vi "multipliers.vi"(7 "LabVIEW Web Service Request":refnum<class "Web Request.lvclass">, 11 "mult":string) -> ()   [LabVIEW 2014]
uses:
  <vilib>/wsapi/Web Request.lvclass
  Controller/Controller.lvclass
  Controller/Messages/Update TE Tech Heating Params/Update TE Tech Heating Params.lvclass
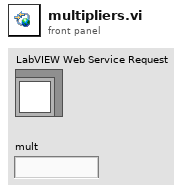
[diagram p1: front panel]
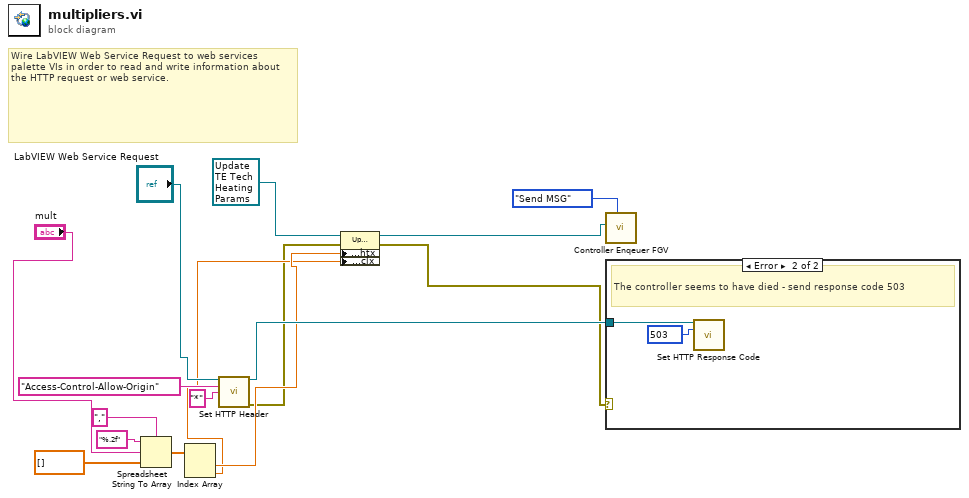
[diagram p0: block diagram]
diagram:
  # "Wire LabVIEW Web Service Request to web services palette VIs in order to read and write information about the HTTP request or web service."
  n1 = Spreadsheet String To Array(delimiter (Tab)=",", format string="%.2f", spreadsheet string="mult", array type (2D Dbl)=dbl[] []) -> (array=w7:dbl[])
  n2 = Index Array(array=w7) -> (element #1=w6:dbl, element #2=w5:dbl)  [unwired: 2 in]
  n3 = call <vilib>:"Set HTTP Header.vi"("LabVIEW Web Service Request"="LabVIEW Web Service Request", "header"="Access-Control-Allow-Origin", "header value"="*") -> ("LabVIEW Web Service Request out"=w14:refnum<class "Web Request.lvclass">, "error out"=w4:errorcluster)  [unwired: 11 in]
  n4 = property class="Update TE Tech Heating Params.l"(reference=refnum<class "Update TE Tech Heating Params.lvclass"> refnum ("Controller:Update TE Tech Heating Params.lvclass"), error in=w4, "Accessors:htx"=w6, "Accessors:clx"=w5) -> (reference out=w2:refnum<class "Update TE Tech Heating Params.lvclass">, error out=w1:errorcluster)
  n5 = call "Controller Enqeuer FGV.vi"("State"=enum16{"Store", "Send MSG"}."Send MSG", "MSG"=w2) -> ()  [unwired: 9 in, 1 out]
  n6 = case shown="Error" w1 {
    tunnel: w14 -> [_ w17]
    frame No Error {
    }
    frame Error {
      w18 = 503 items=["100"=100, "101"=101, "200"=200, "201"=201, "202"=202, "203"=203, "204"=204, "205"=205, "206"=206, "300"=300, "301"=301, "302"=302, "303"=303, "304"=304, "305"=305, "306"=306, "307"=307, "400"=400, "401"=401, "402"=402, "403"=403, "404"=404, "405"=405, "406"=406, "407"=407, "408"=408, "409"=409, "410"=410, "411"=411, "412"=412, "413"=413, "414"=414, "415"=415, "416"=416, "417"=417, "500"=500, "501"=501, "502"=502, "503"=503, "504"=504, "505"=505] ("response code (200)")
      # "The controller seems to have died - send response code 503"
      n7 = call <vilib>:"Set HTTP Response Code.vi"("LabVIEW Web Service Request"=w17, "response code (200)"=w18) -> ()  [unwired: 12 in, 2 out]
    }
  }
